vi "ReadData.vi"() -> ()   [LabVIEW 2013]
panel:
  out "Booléen":bool
  in  "stop":bool
  in  "Attente ms":u32(slide) scale=0.0..200.0
  out "Graphe déroulant":dbl(graph)
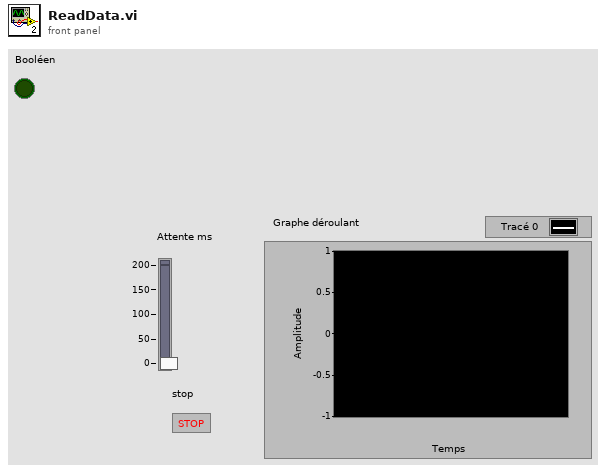
[diagram p1: front panel]
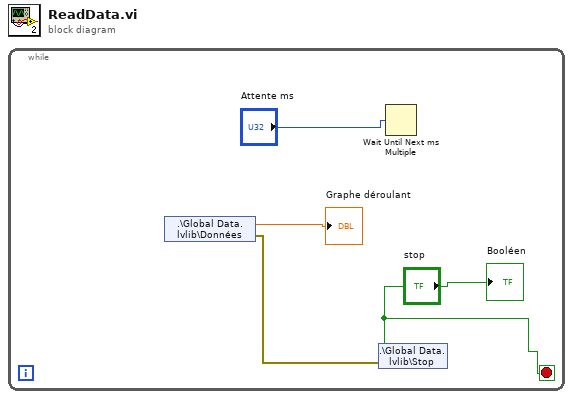
[diagram p0: block diagram]
diagram:
  n1 = while {
    stop <- "stop" stop-if-true
    n2 = shared-variable ".\\Global Data.lvlib\\Données"() -> (→"Graphe déroulant":dbl, error out=w2:errorcluster)  [unwired: 1 in]
    n3 = shared-variable ".\\Global Data.lvlib\\Stop"("stop", error in=w2) -> ()  [unwired: 1 out]
    n4 = Wait Until Next ms Multiple(millisecond multiple="Attente ms") -> ()  [unwired: 1 out]
    "Booléen" <- "stop"
  }
